vi "Get Module Execution Status by ref.vi"(6 "Modules Tree ref":refnum<vi>, 11 "Refs":T1) -> (0 "error out":errorcluster)   [LabVIEW 2023, in "Panther Dashboard.lvlib"]
doc: "This VI checks the Main.vi State of the selected DQMH Module"
uses:
  Panther Dashboard.lvlib
  References Updated Argument--cluster.ctl
  Module type--enum.ctl
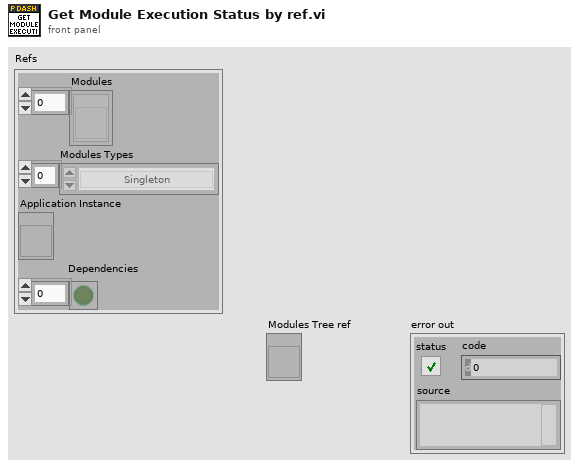
[diagram p1: front panel]
types:
  T1 = typedef "Panther Dashboard.lvlib/References Updated Argument--cluster.ctl" = cluster{"Modules":refnum<vi>[], "Modules Types":T2[], "Application Instance":refnum<vi>, "Dependencies":bool[]}
  T2 = typedef "Panther Dashboard.lvlib/Module type--enum.ctl" = enum16{"Singleton", "Cloneable"}
  T3 = enum32{"Bad", "Idle", "Run top level", "Running"}
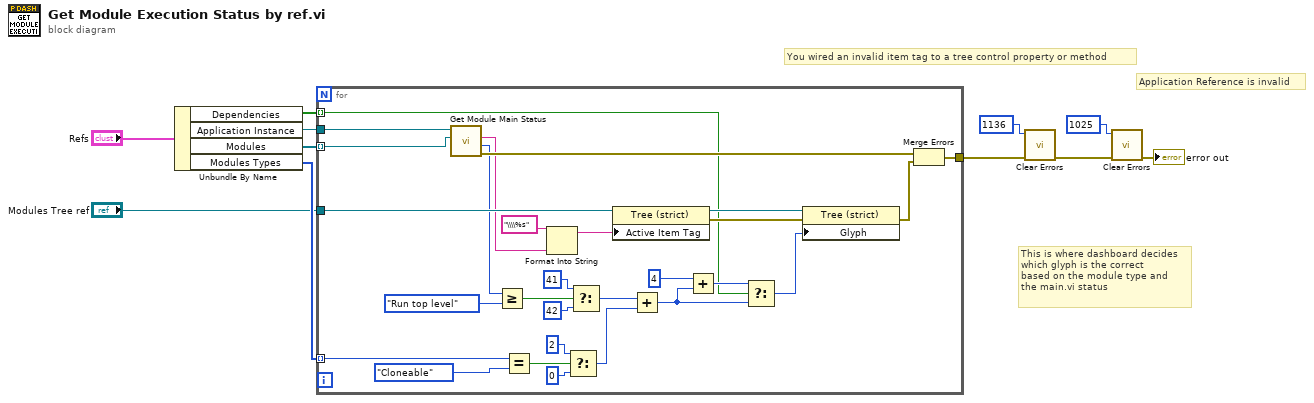
[diagram p0: block diagram]
diagram:
  # "This is where dashboard decides\nwhich glyph is the correct\nbased on the module type and\nthe main.vi status"
  # "Application Reference is invalid"
  # "You wired an invalid item tag to a tree control property or method"
  n1 = Unbundle By Name("Refs") -> ("Dependencies"=w1:bool[], "Application Instance"=w6:refnum<vi>, "Modules"=w5:refnum<vi>[], "Modules Types"=w4:T2[])
  n2 = for {
    tunnel: [w38] -> w11
    tunnel: w5 -> [w18] mode=indexing
    tunnel: "Modules Tree ref" -> [w34]
    tunnel: w4 -> [w26] mode=indexing
    tunnel: w6 -> [w19]
    tunnel: w1 -> [w14] mode=indexing
    n3 = call "Get Module Main Status.vi"("Library in"=w18, "application Instance"=w19) -> ("error out"=w36:errorcluster, "Module Exec State"=w17:T3, "Library Name"=w20:string)  [unwired: 7 in]
    n4 = Greater Or Equal?(x=w17, y=T3."Run top level") -> (x >= y?=w29:bool)
    n5 = Equal?(x=w26, y=Module_type--enum."Cloneable" ("x")) -> (x = y?=w24:bool)
    n6 = Format Into String(format string="\\\\%s", w20) -> (resulting string=w33:string)  [unwired: 2 in, 1 out]
    n7 = Select(t=2, s=w24, f=0) -> (s? t:f=w21:i32)
    n8 = Select(t=41, s=w29, f=42) -> (s? t:f=w31:i32)
    n9 = property class="Tree (strict)"(reference=w34, "Active Item Tag"=w33) -> (reference out=w32:refnum<vi>, error out=w39:errorcluster)  [unwired: 1 in]
    n10 = Add(x=w31, y=w21) -> (x+y=w13:i32)
    n11 = Add(x=4 ("y"), y=w13) -> (x+y=w15:i32)
    n12 = Select(t=w15, s=w14, f=w13) -> (s? t:f=w12:i32)
    n13 = property class="Tree (strict)"(reference=w32, error in=w39, "Glyph"=w12) -> (error out=w37:errorcluster)  [unwired: 1 out]
    n14 = Merge Errors(w36, w37) -> (w38:errorcluster)
  }
  n15 = call <vilib>:"Clear Errors.vi"("error in (no error)"=w11, "specific error code to clear (0: all)"=1136) -> ("error out"=w10:errorcluster)  [unwired: 4 in, 1 out]
  n16 = call <vilib>:"Clear Errors.vi"("error in (no error)"=w10, "specific error code to clear (0: all)"=1025) -> ("error out"=→"error out":errorcluster)  [unwired: 4 in, 1 out]
